vi "Mouse Initialize.vi"(8 "error in (no error)":errorcluster, 11 "UI_Top_Customer in":refnum<class "UI_Top_Customer.lvclass">) -> (0 "error out":errorcluster, 3 "UI_Top_Customer out":refnum<class "UI_Top_Customer.lvclass">)   [LabVIEW 2021, in "UI_Top_Customer.lvclass"]
uses:
  UI_Top_Customer.lvclass
  UI_Top_Customer.lvclass/UI_Top_Customer.ctl
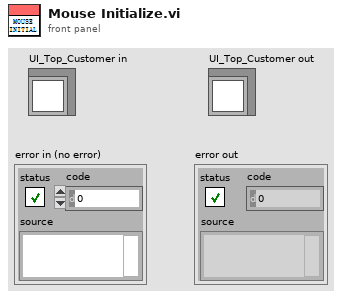
[diagram p1: front panel]
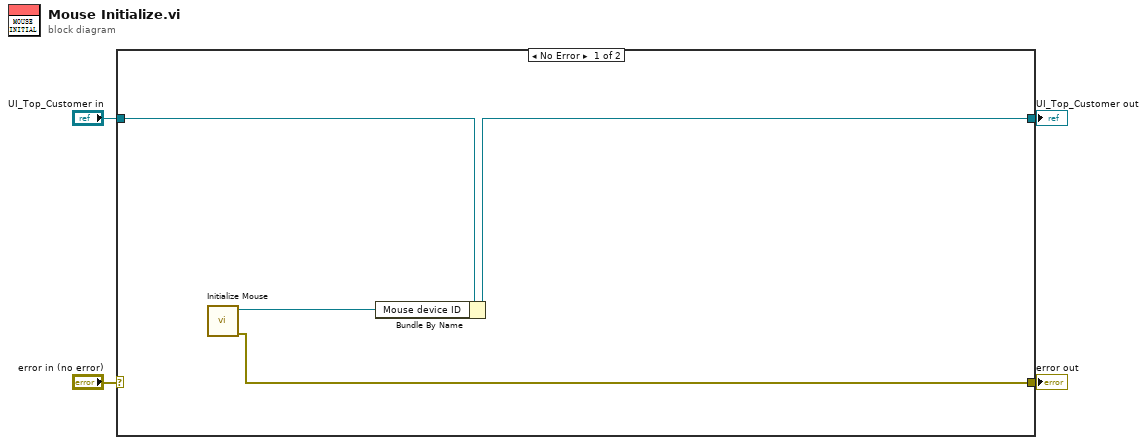
[diagram p0: block diagram]
diagram:
  n1 = case shown="No Error" "error in (no error)" {
    selector: "error in (no error)" -> [_ w10]
    tunnel: [w5 w10] -> w3
    tunnel: [w7 w9] -> w1
    tunnel: "UI_Top_Customer in" -> [w8 w9]
    frame No Error {
      n2 = call <vilib>:"Initialize Mouse.vi"() -> ("error out"=w5:errorcluster, "device ID"=w6:refnum<k1>)  [unwired: 10 in]
      n3 = Bundle By Name(cluster=w8, "Mouse device ID"=w6) -> (w7:refnum<class "UI_Top_Customer.lvclass">)
    }
    frame Error {
    }
  }
  "error out" <- w3
  "UI_Top_Customer out" <- w1
